vi "LCR_Readout.vi"(8 "error in (no error)":errorcluster, 10 "Frequency in Hz":i32, 11 "HP4284A in":refnum<class "HP4284A.lvclass">) -> (0 "error out":errorcluster, 1 "Resistance in Ohm":dbl, 2 "Capacitance in pF":dbl, 3 "HP4284A out":refnum<class "HP4284A.lvclass">)   [LabVIEW 2018, in "HP4284A.lvclass"]
uses:
  HP4284A.lvclass
  LCRControl.lvclass
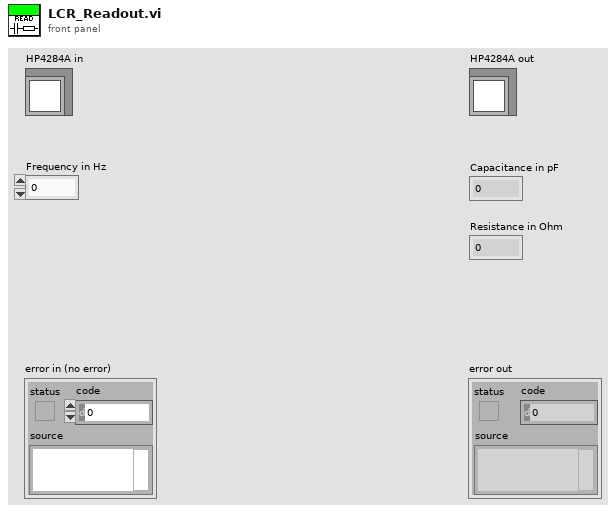
[diagram p1: front panel]
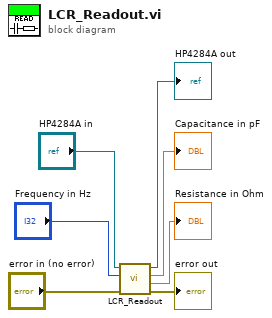
[diagram p0: block diagram]
diagram:
  n1 = call-parent "LCR_Readout.vi"("error in (no error)"="error in (no error)", "Frequency in Hz"="Frequency in Hz", "LCRControl in"="HP4284A in") -> ("error out"=→"error out":errorcluster, "Resistance in Ohm"=→"Resistance in Ohm":dbl, "Capacitance in pF"=→"Capacitance in pF":dbl, "LCRControl out"=→"HP4284A out":refnum<class "HP4284A.lvclass">)  [unwired: 5 in]
